vi "Update.vi"(7 "Value":dbl, 10 "Index":i32, 11 "Variables in":refnum<class "Variables.lvclass">) -> (3 "Variables out":refnum<class "Variables.lvclass">)   [LabVIEW 2020, in "VolatusSeq.lvlib" / "Variables.lvclass"]
uses:
  Variables.lvclass
  Variables.lvclass/Variables.ctl
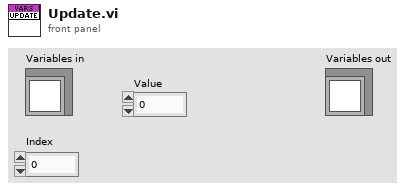
[diagram p1: front panel]
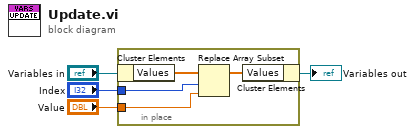
[diagram p0: block diagram]
diagram:
  n1 = in-place {
    in-place-border: "Index" -> [w7]
    in-place-border: "Value" -> [w6]
    n2 = in-place-cluster #1("Variables in") -> ("Values"=w8:dbl[])
    n3 = Replace Array Subset(array=w8, new element=w6, index=w7) -> (w5:dbl[])
    n4 = in-place-cluster #1("Values"=w5) -> (→"Variables out":refnum<class "Variables.lvclass">)
  }
